vi "Replacing The Heart - Lesson 9.vi"() -> ()   [LabVIEW 2023]
doc: "This lesson uses malleable VIs and LabVIEW classes to demonstrate parameterization of the function. This lesson shows a <b>bad idea</b> and why you should be cautious with this approach."
uses:
  Person Information.ctl
  People By Month Wrapper/People By Month Wrapper.lvclass/People By Month Wrapper.ctl
  791c92dc-b78f-4473-b048-a19d6874acda.vi
  45d1eefa-c392-4e6e-b1eb-d27fc55e6400.vi
  b0cddedf-f79d-4358-86cb-e9457ff97cbf.vi
  People By Month Wrapper/Write Person.vi
  People By Month Wrapper/Read Person.vi
  People By Month Wrapper/Less Than.vi
  People By Month Wrapper/People By Month Wrapper.lvclass
panel:
  in  "Starting Month":u16(ring) items=["January", "February", "March", "April", "May", "June", "July", "August", "September", "October", "November", "December"]
  in  "Stop":bool
  out "Sorted People":T1[](array[typedef]) {"Birth Date" format="%<%Y/%b/%d>T"}
  in  "Unsorted People":T1[](array[typedef])=[{"ID"=0, "Family Name"="Tennant", "Given Name"="David", "Birth Date"=timestamp(-6434737636.184167 s since 1904-01-01)}, {"ID"=1, "Family Name"="Smith", "Given Name"="Matt", "Birth Date"=timestamp(-6434726400 s since 1904-01-01)}, {"ID"=2, "Family Name"="Li", "Given Name"="Jing", "Birth Date"=timestamp(3091380833.9038334 s since 1904-01-01)}, {"ID"=3, "Family Name"="Patel", "Given Name"="Aadhya", "Birth Date"=timestamp(3093541462.901833 s since 1904-01-01)}, {"ID"=4, "Family Name"="Doe", "Given Name"="Jane", "Birth Date"=timestamp(3154453586.3918333 s since 1904-01-01)}, {"ID"=5, "Family Name"="Rahman", "Given Name"="Mohammed", "Birth Date"=timestamp(3024418078.500833 s since 1904-01-01)}] {"Birth Date" format="%<%Y/%b/%d>T"}
  # "Overview: As with the functors seen in Lesson 5, doing parameterization with these wrappers seems easy. By supplying an initialization function, we can supply the data to the wrapper. \n\nThis is sometimes fine, but this lesson is going to show you a case where it is a bad idea. Because we are supplying the data as part of each element in the array instead of as a side-function, we have two problems: \n1. We have to be certain that every element of the array is parameterized the same way.\n2. We duplicate the parameterization data into every element, potentially wasting a lot of memory.\n\nThe diagram will explain the problem in greater detail.\n\nInstructions:\n1. Run the VI. As it runs, change the Starting Month. The people will be sorted by birthday but with the people nearest that month prioritized.\n2. Look at the block diagram to see how the sort is done.\n3. Proceed to the next lesson."
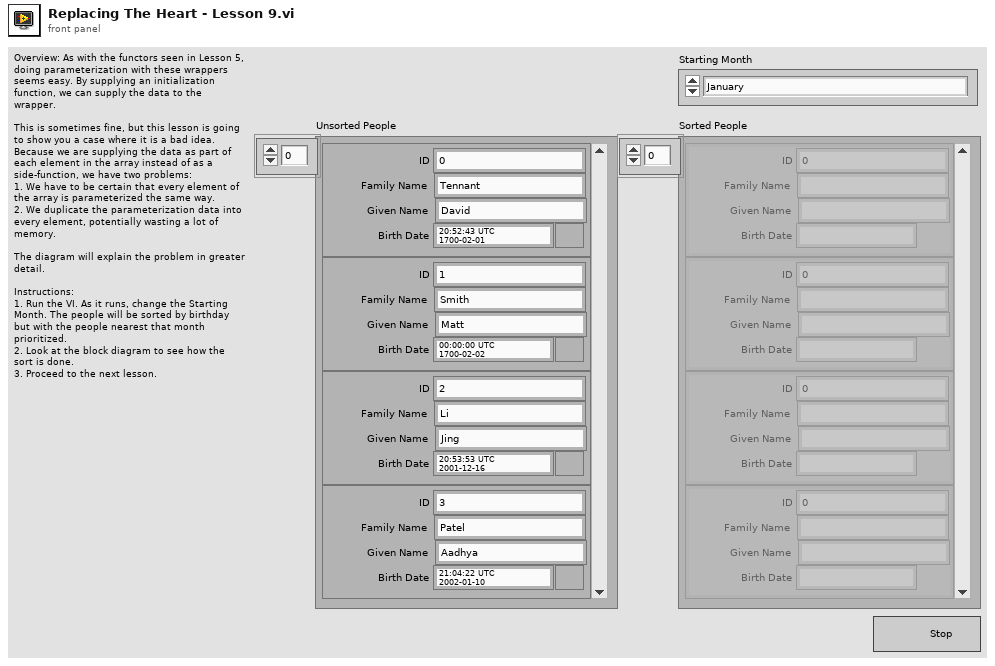
[diagram p1: front panel]
types:
  T1 = typedef "Person Information.ctl" = cluster{"ID":u32, "Family Name":string, "Given Name":string, "Birth Date":timestamp}
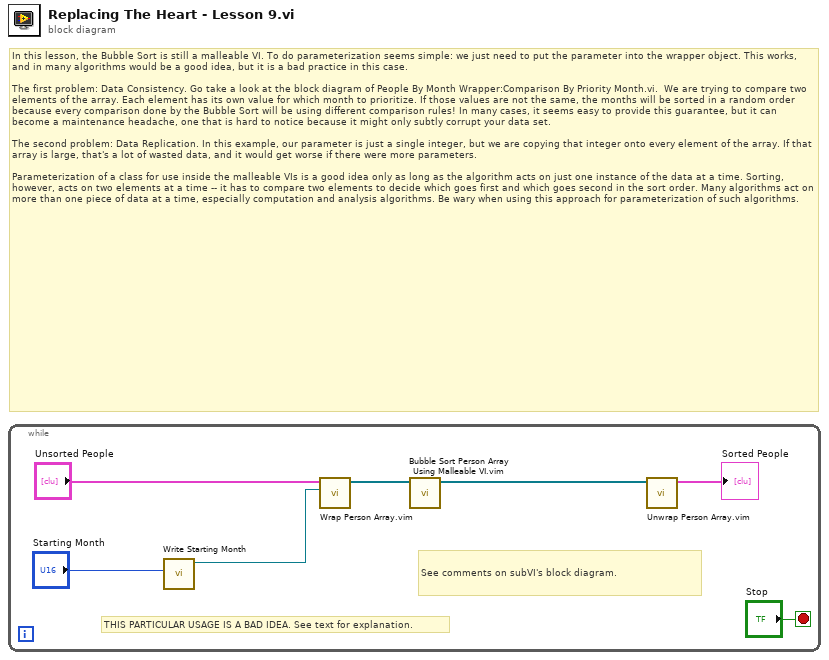
[diagram p0: block diagram]
diagram:
  # "In this lesson, the Bubble Sort is still a malleable VI. To do parameterization seems simple: we just need to put the parameter into the wrapper object. This works, and in many algorithms would be a good idea, but it is a bad practice in this case.\n\nThe first problem: Data Consistency. Go take a look at the block diagram of People By Month Wrapper:Comparison By Priority Month.vi.  We are trying to compare two elements of the array. Each element has its own value for which month to prioritize. If those values are not the same, the months will be sorted in a random order because every comparison done by the Bubble Sort will be using different comparison rules! In many cases, it seems easy to provide this guarantee, but it can become a maintenance headache, one that is hard to notice because it might only subtly corrupt your data set.\n\nThe second problem: Data Replication. In this example, our parameter is just a single integer, but we are copying that integer onto every element of the array. If that array is large, that's a lot of wasted data, and it would get worse if there were more parameters. \n\nParameterization of a class for use inside the malleable VIs is a good idea only as long as the algorithm acts on just one instance of the data at a time. Sorting, however, acts on two elements at a time -- it has to compare two elements to decide which goes first and which goes second in the sort order. Many algorithms act on more than one piece of data at a time, especially computation and analysis algorithms. Be wary when using this approach for parameterization of such algorithms."
  n1 = while {
    stop <- "Stop" stop-if-true
    # "THIS PARTICULAR USAGE IS A BAD IDEA. See text for explanation."
    # "See comments on subVI's block diagram."
    n2 = call "Write Starting Month.vi"("Starting Month"="Starting Month") -> ("People By Month Wrapper out"=w1:refnum<class "People By Month Wrapper.lvclass">)  [unwired: 10 in]
    n3 = call "Wrap Person Array.vim"("People Wrapper in"=w1, "Unsorted People"="Unsorted People") -> ("Array"=w6:refnum<class "People By Month Wrapper.lvclass">[])  [unwired: 9 in]
    n4 = call "Bubble Sort Person Array Using Malleable VI.vim"("Unsorted"=w6) -> ("Sorted"=w4:refnum<class "People By Month Wrapper.lvclass">[])  [unwired: 10 in]
    n5 = call "Unwrap Person Array.vim"("Sorted"=w4) -> ("Array"=→"Sorted People":T1[])  [unwired: 10 in]
  }
